vi "_Get Interfaces.vi"(8 "error in (no error)":errorcluster, 11 "CellPhone in":refnum<class "CellPhone.lvclass">) -> (0 "error out":errorcluster, 2 "Concrete Interfaces":refnum<class "IUnknown.lvclass">[](array[class]), 3 "CellPhone out":refnum<class "CellPhone.lvclass">)   [LabVIEW 2009, in "CellPhone.lvclass"]
doc: "Returns an array of Interfaces the object has implemented. Child classes must override this vi."
uses:
  CellPhone.lvclass
  Source/IUnknown Class/IUnknown.lvclass
  ISleepableCellPhone/ISleepableCellPhone.lvclass
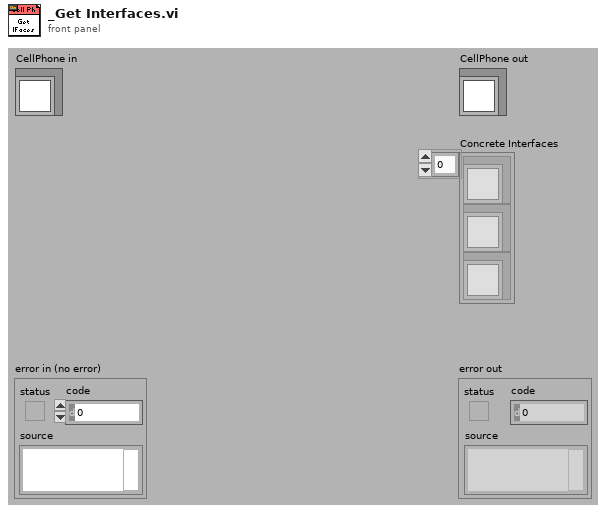
[diagram p1: front panel]
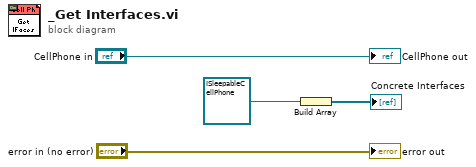
[diagram p0: block diagram]
diagram:
  n1 = Build Array(refnum<class "ISleepableCellPhone.lvclass"> refnum ("CellPhone ISleepable")) -> (→"Concrete Interfaces":refnum<class "ISleepableCellPhone.lvclass">[])
  "error out" <- "error in (no error)"
  "CellPhone out" <- "CellPhone in"
